vi "ExportConfigurationToFile.vi"(8 "error in (no error)":errorcluster, 11 "Node Ptr":u64 format="%.0x") -> (0 "error out":errorcluster)   [LabVIEW 2019, in "Instrument Addon System Explorer.lvlib"]
uses:
  Instrument Addon System Explorer.lvlib
  <vilib>/NI/GXML/GXML.lvlib
  <vilib>/NI VeriStand/Custom Device API/Custom Device API.lvlib
  <vilib>/NI/NI VeriStand Custom Device Import and Export Tool/ImportExport.lvlib
panel:
  in  "Tag":string
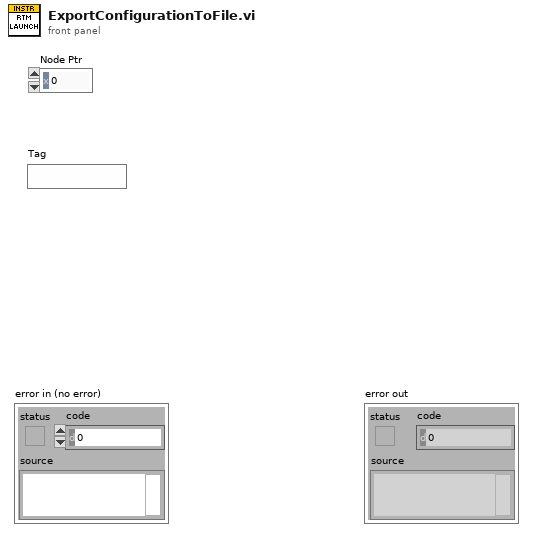
[diagram p1: front panel]
types:
  T1 = typedef "Custom Device API.lvlib/Custom Device Item Ref.ctl" = u64
  T2 = typedef "Instrument Addon System Explorer.lvlib/Instrument Custom Device SysDef Configuration V1.0.1.ctl" = cluster{"Name":string, "Description":string, "Protocol":string, "RS232 Config":T3, "MetaData Globals":T4[], "Message Groups":T11[], "GPIB Config":T25, "TCPIP Config":T26, "Decimation":u32, "UDP Config":T27}
  T3 = typedef "Instrument Addon Shared.lvlib/RSXXX Port Settings.ctl" = cluster{"Port":string, "Baud Rate":u32, "Data Bits":u16, "Parity":enum16{"None", "Odd", "Even", "Mark", "Space"}, "Stop Bits":u16, "Flow Control":u16, "XON":enum16{"NUL", "SOH", "STX", "ETX", "EOT", "ENQ", "ACK", "BEL", "BS", "HT", "LF", "VT", "FF", "CR", "SO", "SI", "DLE", "DC1", "DC2", "DC3", "DC4", "NAK", "SYN", "ETB", "CAN", "EM", "SUB", "ESC", "FS", "GS", "RS", "US", "SP", "!", "\"", "#", "$", "%", "&", "'", "(", ")", "*", "+", ",", "- (-)", ".", "/", "0", "1", "2", "3", "4", "5", "6", "7", "8", "9", ":", ";", "<", "=", ">", "?", "@", "A", "B", "C", "D", "E", "F", "G", "H", "I", "J", "K", "L", "M", "N", "O", "P", "Q", "R", "S", "T", "U", "V", "W", "X", "Y", "Z", "[", "\\", "]", "^", "_", "`", "a", "b", "c", "d", "e", "f", "g", "h", "i", "j", "k", "l", "m", "n", "o", "p", "q", "r", "s", "t", "u", "v", "w", "x", "y", "z", "{", "|", "}", "~"}, "XOFF":enum16{"NUL", "SOH", "STX", "ETX", "EOT", "ENQ", "ACK", "BEL", "BS", "HT", "LF", "VT", "FF", "CR", "SO", "SI", "DLE", "DC1", "DC2", "DC3", "DC4", "NAK", "SYN", "ETB", "CAN", "EM", "SUB", "ESC", "FS", "GS", "RS", "US", "SP", "!", "\"", "#", "$", "%", "&", "'", "(", ")", "*", "+", ",", "- (-)", ".", "/", "0", "1", "2", "3", "4", "5", "6", "7", "8", "9", ":", ";", "<", "=", ">", "?", "@", "A", "B", "C", "D", "E", "F", "G", "H", "I", "J", "K", "L", "M", "N", "O", "P", "Q", "R", "S", "T", "U", "V", "W", "X", "Y", "Z", "[", "\\", "]", "^", "_", "`", "a", "b", "c", "d", "e", "f", "g", "h", "i", "j", "k", "l", "m", "n", "o", "p", "q", "r", "s", "t", "u", "v", "w", "x", "y", "z", "{", "|", "}", "~"}, "End Read on Termination Character":bool, "End Write on Termination Character":bool, "Termination Character":u8}
  T4 = typedef "Instrument Addon System Explorer.lvlib/MetaData Channel Configuration.ctl" = cluster{"Name":string, "Description":string, "MetaData Parameters":T5, "Config GUID":string, "Channel Array":T10[]}
  T5 = typedef "Instrument Addon Shared.lvlib/MetaData Parameters.ctl" = cluster{"Data Type":T6, "Channel Type":T7, "List":string[], "Format String":string, "Type":T8, "Delimiter":string, "Endian":T9}
  T6 = typedef "Instrument Addon Shared.lvlib/Protocol Data Type.ctl" = enum16{"Single Channel", "Array"}
  T7 = typedef "Instrument Addon Shared.lvlib/Metadata Channel Type.ctl" = enum16{"Enumerated List", "Format", "Type Cast"}
  T8 = typedef "Instrument Addon Shared.lvlib/Type Cast Type.ctl" = enum16{"DBL", "SGL", "U64", "U32", "U16", "U8", "I64", "I32", "I16", "I8"}
  T9 = typedef "Instrument Addon Shared.lvlib/Endian.ctl" = enum16{"Native", "Little", "Big"}
  T10 = typedef "Instrument Addon System Explorer.lvlib/Channel Properties.ctl" = cluster{"Name":string, "Units":string, "Default Value":dbl}
  T11 = typedef "Instrument Addon System Explorer.lvlib/Message Group Configuration.ctl" = cluster{"Name":string, "Description":string, "Messages":T12[]}
  T12 = typedef "Instrument Addon System Explorer.lvlib/Message Configuration.ctl" = cluster{"Name":string, "Description":string, "Command":T13, "Response":T16, "Message Settings":T22, "Periodic Enabled":dbl, "Trigger Parameters":T24}
  T13 = typedef "Instrument Addon System Explorer.lvlib/Command Message Configuration.ctl" = cluster{"Description":string, "Command Parameters":T14, "MetaData Channels":T4[]}
  T14 = typedef "Instrument Addon Shared.lvlib/Command Parameters.ctl" = cluster{"Command":string, "Linked Channels":T15[], "Pad":bool, "Length":u32, "Pad Value":u8}
  T15 = typedef "Instrument Addon Shared.lvlib/Linked Channel Cluster.ctl" = cluster{"Variable Name":string, "GUID":string}
  T16 = typedef "Instrument Addon System Explorer.lvlib/Response Message Configuration.ctl" = cluster{"Description":string, "Reponse Parameters":T17, "Data Channels":T19[]}
  T17 = typedef "Instrument Addon Shared.lvlib/Response Parameters.ctl" = cluster{"Response":string, "Linked Channels":T15[], "Type Value":dbl, "Wait Type":T18, "Use Channel":bool, "Channel Path":string}
  T18 = typedef "Instrument Addon Shared.lvlib/Response Wait Type.ctl" = enum16{"Byte Count", "Wait sec"}
  T19 = typedef "Instrument Addon System Explorer.lvlib/Data Channel Configuration.ctl" = cluster{"Name":string, "Description":string, "Data Parameters":T20, "Config GUID":string, "Channel Array":T10[]}
  T20 = typedef "Instrument Addon Shared.lvlib/Data Parameters.ctl" = cluster{"Data Type":T6, "Channel Type":T21, "Format String":string, "Expected String":string, "Type":T8, "List":string[], "Delimiter":string, "Endian":T9}
  T21 = typedef "Instrument Addon Shared.lvlib/Data Channel Type.ctl" = enum16{"Format", "Comparison", "Type Cast", "Enumerated List"}
  T22 = typedef "Instrument Addon Shared.lvlib/Message Parameters.ctl" = cluster{"Generation Type":T23, "Period":dbl, "Include Protection":bool, "Type":string}
  T23 = typedef "Instrument Addon Shared.lvlib/Message Generation Type.ctl" = enum16{"Trigger Only", "Periodic & Trigger", "Value Change & Trigger"}
  T24 = typedef "Instrument Addon Shared.lvlib/Trigger Parameters.ctl" = cluster{"Use Channel":bool, "Channel Path":string}
  T25 = typedef "Instrument Addon Shared.lvlib/VISA Settings.ctl" = cluster{"VISA Resource":string, "Enable Termination Character":bool, "Termination Character":u8, "Timeout":u32, "Append Write Termination Character":bool}
  T26 = typedef "Instrument Addon Shared.lvlib/TCPIP Settings.ctl" = cluster{"IP Address":string, "Port":u16}
  T27 = typedef "Instrument Addon Shared.lvlib/UDP Settings.ctl" = cluster{"Local IP Address":string, "Local Port":u16, "Target IP Address":string, "Target Port":u16}
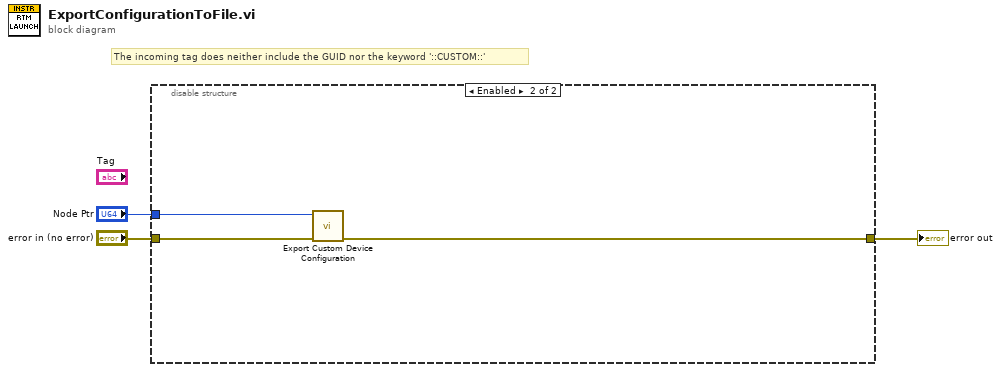
[diagram p0: block diagram]
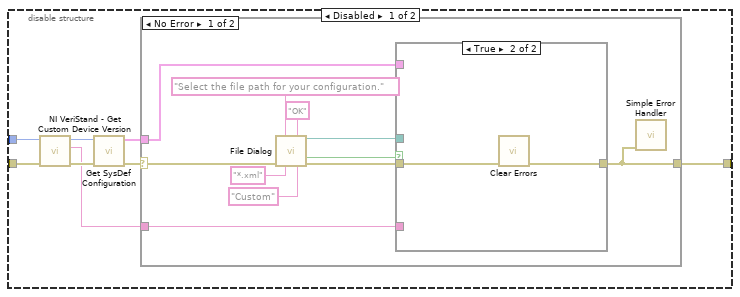
[diagram p2: hidden frame]
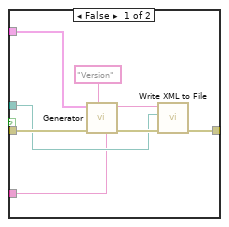
[diagram p3: hidden frame]
diagram:
  # "The incoming tag does neither include the GUID nor the keyword '::CUSTOM::'"
  n1 = disable-structure shown="Enabled" {
    disable-tunnel: "Node Ptr" -> [w9 w35]
    disable-tunnel: "error in (no error)" -> [w7 w36]
    disable-tunnel: [w4 w34] -> w1
    frame Disabled {
      n2 = call <vilib>:"NI VeriStand - Get Custom Device Version.vi"("error in (no error)"=w7, "Device Ref in"=w9) -> ("error out"=w6:errorcluster, "Value"=w5:string, "Device Ref out"=w8:T1)  [unwired: 7 in]
      n3 = call "Get SysDef Configuration.vi"("error in (no error)"=w6, "Node Ptr"=w8) -> ("error out"=w11:errorcluster, "Configuration"=w10:T2)  [unwired: 8 in]
      n4 = case shown="No Error" w11 {
        selector: w11 -> [w18 w33]
        tunnel: [w12 w33] -> w4
        tunnel: w10 -> [w14 _]
        tunnel: w5 -> [w13 _]
        frame No Error {
          n5 = call "File Dialog"("prompt"="Select the file path for your configuration.", "button label"="OK", "error in"=w18, "pattern (all files)"="*.xml", "pattern label"="Custom") -> ("selected path"=w15:path, "cancelled"=w17:bool, "error out"=w16:errorcluster)  [unwired: 7 in, 1 out]
          n6 = case shown="True" w17 {
            tunnel: [w27 w31] -> w12
            tunnel: w16 -> [w26 w32]
            tunnel: w15 -> [w25 _]
            tunnel: w14 -> [w24 _]
            tunnel: w13 -> [w23 _]
            frame False {
              n7 = call <vilib>:"Generator.vi"("Version String"=w23, "Version Tag Name"="Version", "error in"=w26, "Variant"=w24) -> ("error out"=w28:errorcluster, "XML String Out"=w30:string)  [unwired: 6 in]
              n8 = call <vilib>:"Write XML to File.vi"("error in"=w28, "XML File Path"=w25, "XML Input"=w30) -> ("error out"=w27:errorcluster)  [unwired: 8 in]
            }
            frame True {
              n9 = call <vilib>:"Clear Errors.vi"("error in (no error)"=w32) -> ("error out"=w31:errorcluster)  [unwired: 5 in, 1 out]
            }
          }
          n10 = call <vilib>:"Simple Error Handler.vi"("error in (no error)"=w12) -> ()  [unwired: 4 in, 5 out]
        }
        frame Error {
        }
      }
    }
    frame Enabled {
      n11 = call <vilib>:"Export Custom Device Configuration.vi"("error in (no error)"=w36, "ID"=w35) -> ("error out"=w34:errorcluster)  [unwired: 8 in, 1 out]
    }
  }
  "error out" <- w1
